vi "readtdms.vi"   [LabVIEW 2014]
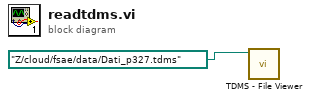
[diagram p0: block diagram]
diagram:
  n1 = call <vilib>:"TDMS - File Viewer.vi"("file path"=path "Z:/cloud/fsae/data/Dati_p327.tdms") -> ()  [unwired: 5 in, 2 out]
